vi "OneSessTwoPinOneSystemPinOneInstrOneSiteReservation_CallGetConnectionsFromPinsForTwoDcPowerPinsAllSites_ReturnsTwoConnections.vi"(8 "error in":errorcluster) -> (0 "error out":errorcluster, 2 "result":string, 3 "pass":bool)   [LabVIEW 2020, in "MeasurementServerTests.lvlib"]
uses:
  MeasurementServerTests.lvlib
  Runtime/MeasurementLink Session Management/Session Reservation/Connection with Session.ctl
  Runtime/MeasurementLink Session Management/Session Reservation/Connection.ctl
  Runtime/MeasurementLink niDCPower/Instrument/Instrument.lvclass
  C:/dev/measurementlink-labview/Source/Runtime/MeasurementLink Instrument/IInstrument/IInstrument.lvclass
  54d890a8-4121-421c-bfc5-08266fe71a04.vi
  777eb16d-c0be-4c50-a7a6-d4611c66469e.vi
  c3cb69a0-23cd-49fc-99d1-8c54773f0200.vi
  b3e5c3be-b7a7-4b6e-86ee-709eea9cb752.vi
  Runtime/MeasurementLink Session Management/Session Reservation/Get Connections Impl.vi
  Runtime/MeasurementLink Session Management/Session Reservation/Session Reservation.lvclass
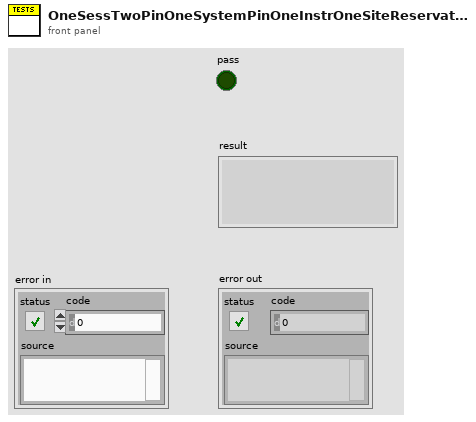
[diagram p1: front panel]
types:
  T1 = typedef "MeasurementLink Session Management.lvlib/Session Reservation.lvclass/Connection.ctl" = cluster{"pin or relay name":string, "site":i32, "instrument type id":string, "channel":string}
  T2 = typedef "MeasurementLink Session Management.lvlib/Session Reservation.lvclass/Connection with Session.ctl" = cluster{"connection":T1, "session":variant}
  T3 = typedef "MeasurementLink Session Management.lvlib/Session Reservation.lvclass/Data.ctl" = cluster{"session and driver infos":T4[], "pin or relay names":string[], "connection map":refnum<class "Connection Map.lvclass">, "pin map context":T8}
  T4 = typedef "MeasurementLink Session Management.lvlib/Session Reservation.lvclass/Session and Driver Info.ctl" = cluster{"session info":T5, "session":variant}
  T5 = typedef "MeasurementLink Session Management Client.lvlib/ni_measurementlink_sessionmanagement_v1_SessionInformation.ctl" = cluster{"session":T6, "resource_name":string, "channel_list":string, "instrument_type_id":string, "session_exists":bool, "channel_mappings":T7[]}
  T6 = typedef "MeasurementLink Session Management Client.lvlib/nidevice_grpc_Session.ctl" = cluster{"name":string}
  T7 = typedef "MeasurementLink Session Management Client.lvlib/ni_measurementlink_sessionmanagement_v1_ChannelMapping.ctl" = cluster{"pin_or_relay_name":string, "site":i32, "channel":string}
  T8 = typedef "MeasurementLink Session Management Client.lvlib/ni_measurementlink_PinMapContext.ctl" = cluster{"pin_map_id":string, "sites":i32[]}
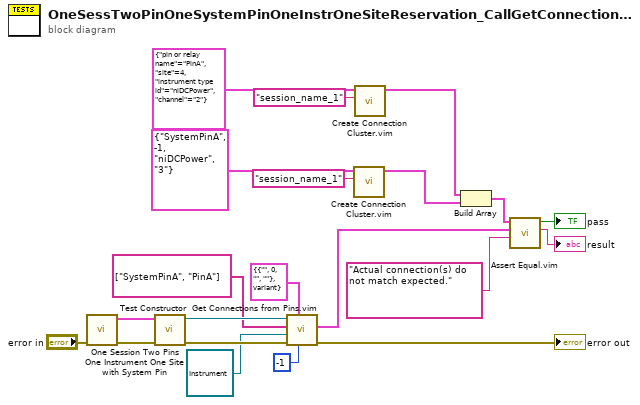
[diagram p0: block diagram]
diagram:
  n1 = call "One Session Two Pins One Instrument One Site with System Pin.vi"("error in"="error in") -> ("error out"=w11:errorcluster, "data out"=w10:T3)  [unwired: 9 in]
  n2 = call "Test Constructor.vi"("error in"=w11, "data"=w10) -> ("error out"=w20:errorcluster, "Session Reservation out"=w19:refnum<class "Session Reservation.lvclass">)  [unwired: 8 in]
  n3 = call "Get Connections from Pins.vim"("site"=-1, "connection type"=T2 {"connection"={"pin or relay name"="", "site"=0, "instrument type id"="", "channel"=""}, "session"=variant} ("connection"), "error in"=w20, "instrument"=refnum<class "Instrument.lvclass"> refnum ("MeasurementLink niDCPower.lvlib:Instrument.lvclass"), "pin or relay names"=string[] ["SystemPinA", "PinA"], "session reservation in"=w19) -> ("error out"=→"error out":errorcluster, "connections"=w16:T2[])  [unwired: 3 in, 1 out]
  n4 = call "Create Connection Cluster.vim"("session in"="session_name_1", "hardware independent connection in"=T1 {"pin or relay name"="SystemPinA", "site"=-1, "instrument type id"="niDCPower", "channel"="3"} ("connection")) -> ("connection out"=w9:T2)  [unwired: 9 in]
  n5 = call "Create Connection Cluster.vim"("session in"="session_name_1", "hardware independent connection in"=T1 {"pin or relay name"="PinA", "site"=4, "instrument type id"="niDCPower", "channel"="2"} ("connection")) -> ("connection out"=w1:T2)  [unwired: 9 in]
  n6 = Build Array(w1, w9) -> (w8:T2[])
  n7 = call "Assert Equal.vim"("failure message"="Actual connection(s) do not match expected.", "actual value"=w16, "expected value"=w8) -> ("message"=→"result":string, "equal?"=→"pass":bool)  [unwired: 7 in]
